vi "easy stream read.vi"(8 "error in":errorcluster, 9 "Scans To Read":i32=1000, 10 "# Channels In Stream":i32, 11 "Handle In":i32) -> (0 "error out":errorcluster, 1 "Stream Parameters":T1 {"Device Backlog [%]" format="%.2f"}, 2 "Data":dbl[][](array[numeric]) format="%.3f", 3 "Handle Out":i32)   [LabVIEW 2021]
panel:
  # "Pass the number of channels being streamed, not\njust how many you want to read."
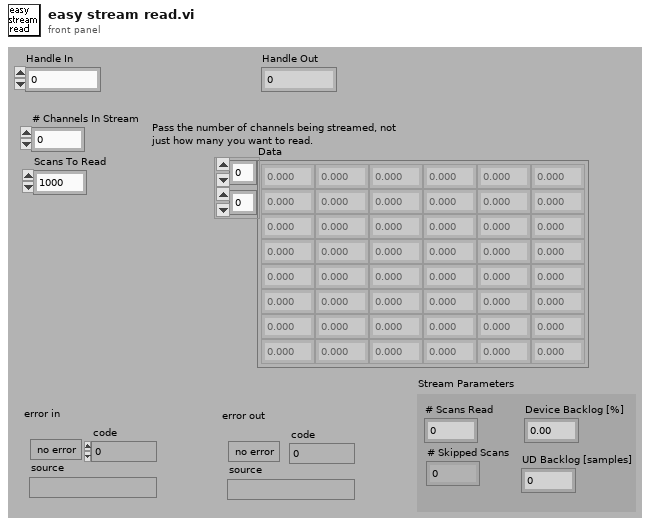
[diagram p1: front panel]
types:
  T1 = cluster{"# Scans Read":i32, "# Skipped Scans":i32, "Device Backlog [%]":dbl, "UD Backlog [samples]":i32}
  T2 = cluster{"# Scans Read":i32, "# Skipped Scans":i32, "U3 Backlog [%]":dbl, "UD Backlog [samples]":i32}
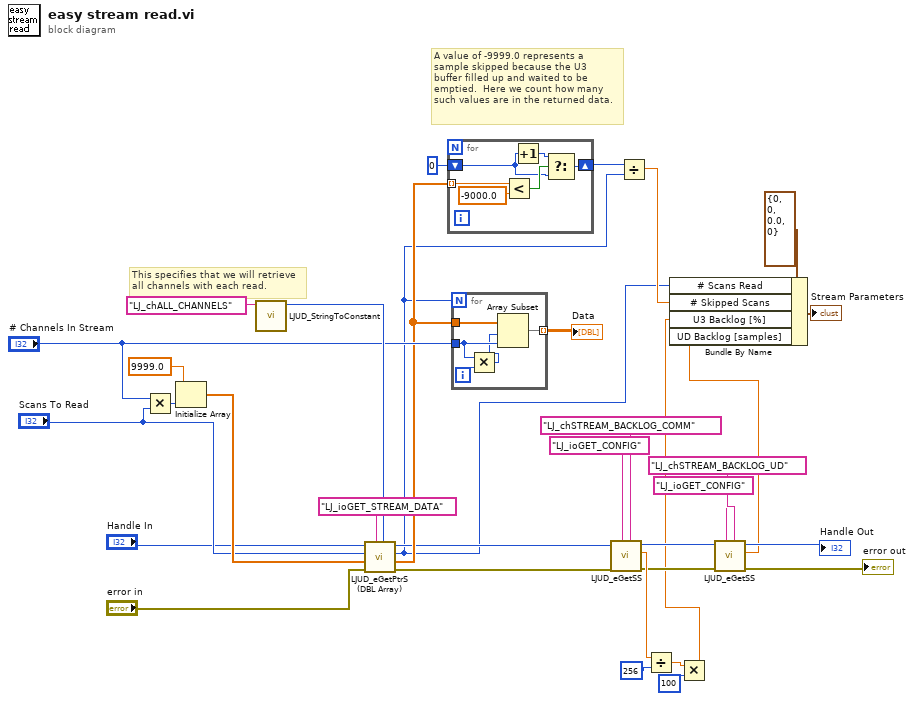
[diagram p0: block diagram]
diagram:
  # "A value of -9999.0 represents a\nsample skipped because the U3\nbuffer filled up and waited to be\nemptied.  Here we count how many\nsuch values are in the returned data."
  # "This specifies that we will retrieve\nall channels with each read."
  n1 = Multiply(x="# Channels In Stream", y="Scans To Read") -> (x*y=w30:i32)
  n2 = Initialize Array(9999.0, w30) -> (w32:dbl[])
  n3 = call "LJUD_StringToConstant.vi"("String"="LJ_chALL_CHANNELS") -> ("Constant Number"=w34:i32)  [unwired: 9 in, 1 out]
  n4 = call "LJUD_eGetPtrS (DBL Array).vi"("Channel"=w34, "IOType"="LJ_ioGET_STREAM_DATA", "error in"="error in", "DBL Array Write"=w32, "Value"="Scans To Read", "Handle In"="Handle In") -> ("error out"=w11:errorcluster, "DBL Array Read"=w9:dbl[], "Value"=w3:i32, "Handle Out"=w8:i32)  [unwired: 2 in]
  n5 = for {
    shift-right: [w35] -> w13
    shift-left: 0 -> [w36]
    tunnel: w9 -> [w39] mode=indexing
    n6 = Less?(x=w39, y=-9000.0) -> (x < y?=w37:bool)
    n7 = Increment(x=w36) -> (x+1=w40:i32)
    n8 = Select(t=w40, s=w37, f=w36) -> (s? t:f=w35:i32)
  }
  n9 = for {
    N: w3 -> [_]
    tunnel: w9 -> [w45]
    tunnel: "# Channels In Stream" -> [w44]
    tunnel: [w41] -> w24 mode=indexing
    i -> [w43]
    n10 = Multiply(x=w44, y=w43) -> (x*y=w42:i32)
    n11 = Array Subset(array=w45, index=w42, length=w44) -> (w41:dbl[])
  }
  "Data" <- w24
  n12 = call "LJUD_eGetSS.vi"("Channel"="LJ_chSTREAM_BACKLOG_COMM", "IOType"="LJ_ioGET_CONFIG", "error in"=w11, "Handle In"=w8) -> ("error out"=w19:errorcluster, "Value Read"=w23:dbl, "Handle Out"=w18:i32)  [unwired: 5 in]
  n13 = Divide(x=w13, y=w3) -> (x/y=w4:dbl)
  n14 = Divide(x=w23, y=256) -> (x/y=w20:dbl)
  n15 = Multiply(x=w20, y=100) -> (x*y=w2:dbl)
  n16 = call "LJUD_eGetSS.vi"("Channel"="LJ_chSTREAM_BACKLOG_UD", "IOType"="LJ_ioGET_CONFIG", "error in"=w19, "Handle In"=w18) -> ("error out"=→"error out":errorcluster, "Value Read"=w1:dbl, "Handle Out"=→"Handle Out":i32)  [unwired: 5 in]
  n17 = Bundle By Name(cluster=T2 {"# Scans Read"=0, "# Skipped Scans"=0, "U3 Backlog [%]"=0.0, "UD Backlog [samples]"=0} ("Stream Parameters"), "# Scans Read"=w3, "# Skipped Scans"=w4, "U3 Backlog [%]"=w2, "UD Backlog [samples]"=w1) -> (→"Stream Parameters":T2)
